vi "SETParametersToSPCdata.vi"(8 "ErrorIn":errorcluster, 10 "setFile":path=path "X:/Jannis/Abgleich/150-n scanin.set", 11 "SPCdataIn":T1={"base_adr"=0, "init"=0, "cfd_limit_low"=0.0, "cfd_limit_high"=0.0, "cfd_zc_level"=0.0, "cfd_holdoff"=0.0, "sync_zc_level"=0.0, "sync_holdoff"=0.0, "sync_threshold"=0.0, "tac_range"=0.0, "sync_freq_div"=0, "tac_gain"=0, "tac_offset"=0.0, "tac_limit_low"=0.0, "tac_limit_high"=0.0, "adc_resolution"=12, "ext_latch_delay"=0, "collect_time"=0.0, "display_time"=0.0, "repeat_time"=0.0, "stop_on_time"=0, "stop_on_ovfl"=0, "dither_range"=0, "count_incr"=0, "mem_bank"=0, "dead_time_comp"=0, "scan_control"=0, "routing_mode"=0, "tac_enable_hold"=0.0, "pci_card_no"=0, "mode"=0, "scan_size_x"=0, "scan_size_y"=0, "scan_rout_x"=0, "scan_rout_y"=0, "scan_flyback"=0, "scan_borders"=0, "scan_polarity"=0, "pixel_clock"=0, "line_compression"=0, "trigger"=0, "pixel_time"=0.0, "ext_pixclk_div"=0, "rate_count_time"=0.0, "macro_time_clk"=0, "add_select"=0, "test_eep"=0, "adc_zoom"=0, "img_size_x"=0, "img_size_y"=0, "img_rout_x"=0, "img_rout_y"=0, "xy_gain"=0, "master_clock"=0, "adc_sample_delay"=0, "detector_type"=0, "chan_enable"=0, "chan_slope"=0, "chan_spec_no"=0, "tdc_control"=0, "tdc_offset1"=0.0, "tdc_offset2"=0.0, "tdc_offset3"=0.0, "tdc_offset4"=0.0, "tdc_offset5"=0.0, "tdc_offset6"=0.0, "cfd_th5_tdc"=0.0, "cfd_th6_tdc"=0.0, "cfd_zc5_tdc"=0.0, "cfd_zc6_tdc"=0.0, "future_reserve1"=0, "future_reserve2"=0, "future_reserve3"=0, "future_reserve4"=0}) -> (0 "ErrorOut":errorcluster, 3 "SPCdataOut":T1={"base_adr"=0, "init"=0, "cfd_limit_low"=0.0, "cfd_limit_high"=0.0, "cfd_zc_level"=0.0, "cfd_holdoff"=0.0, "sync_zc_level"=0.0, "sync_holdoff"=0.0, "sync_threshold"=0.0, "tac_range"=0.0, "sync_freq_div"=0, "tac_gain"=0, "tac_offset"=0.0, "tac_limit_low"=0.0, "tac_limit_high"=0.0, "adc_resolution"=12, "ext_latch_delay"=0, "collect_time"=0.0, "display_time"=0.0, "repeat_time"=0.0, "stop_on_time"=0, "stop_on_ovfl"=0, "dither_range"=0, "count_incr"=0, "mem_bank"=0, "dead_time_comp"=0, "scan_control"=0, "routing_mode"=0, "tac_enable_hold"=0.0, "pci_card_no"=0, "mode"=0, "scan_size_x"=0, "scan_size_y"=0, "scan_rout_x"=0, "scan_rout_y"=0, "scan_flyback"=0, "scan_borders"=0, "scan_polarity"=0, "pixel_clock"=0, "line_compression"=0, "trigger"=0, "pixel_time"=0.0, "ext_pixclk_div"=0, "rate_count_time"=0.0, "macro_time_clk"=0, "add_select"=0, "test_eep"=0, "adc_zoom"=0, "img_size_x"=0, "img_size_y"=0, "img_rout_x"=0, "img_rout_y"=0, "xy_gain"=0, "master_clock"=0, "adc_sample_delay"=0, "detector_type"=0, "chan_enable"=0, "chan_slope"=0, "chan_spec_no"=0, "tdc_control"=0, "tdc_offset1"=0.0, "tdc_offset2"=0.0, "tdc_offset3"=0.0, "tdc_offset4"=0.0, "tdc_offset5"=0.0, "tdc_offset6"=0.0, "cfd_th5_tdc"=0.0, "cfd_th6_tdc"=0.0, "cfd_zc5_tdc"=0.0, "cfd_zc6_tdc"=0.0, "future_reserve1"=0, "future_reserve2"=0, "future_reserve3"=0, "future_reserve4"=0}, 4 "DecayMatrix":cluster{"Waveform Graph":sgl[]}[][](array[cluster]), 5 "ActiveModule":string[](array[string]))   [LabVIEW 2023]
doc: "This VI aids to read a full set of system parameters from a .set-file or the header of a .sdt into the SPCdata cluster. Usefull when wanting to copy all parameters established in SPCM.exe to the LV-environment.\nNote, that some parameters like <b>mode</b> are not mapped. To correctly set these parameters use SPC_set- and get_parameters.vi before calling this VI."
uses:
  SPC_Wrappers/SPC_Controls/Systparm_Kewords.ctl
  SPC_Wrappers/SPC_Controls/SPCdata.ctl
panel:
  out "String":string
  in  "Systparm_Keywords":T2
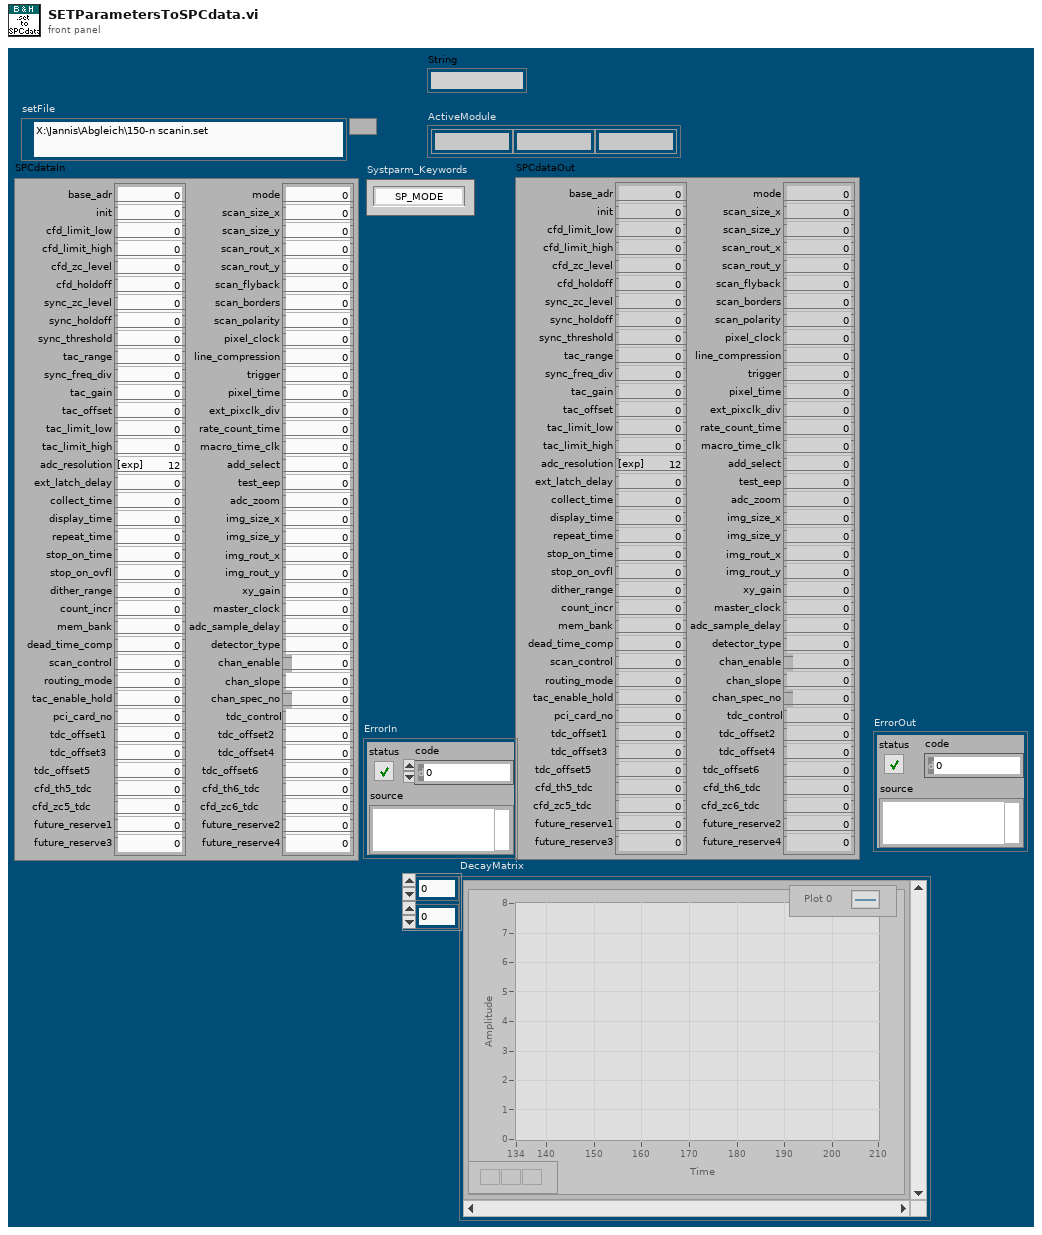
[diagram p1: front panel]
types:
  T1 = typedef "SPCdata.ctl" = cluster{"base_adr":u16, "init":i16, "cfd_limit_low":sgl, "cfd_limit_high":sgl, "cfd_zc_level":sgl, "cfd_holdoff":sgl, "sync_zc_level":sgl, "sync_holdoff":sgl, "sync_threshold":sgl, "tac_range":sgl, "sync_freq_div":i16, "tac_gain":i16, "tac_offset":sgl, "tac_limit_low":sgl, "tac_limit_high":sgl, "adc_resolution":i16, "ext_latch_delay":i16, "collect_time":sgl, "display_time":sgl, "repeat_time":sgl, "stop_on_time":i16, "stop_on_ovfl":i16, "dither_range":i16, "count_incr":i16, "mem_bank":i16, "dead_time_comp":i16, "scan_control":u16, "routing_mode":u16, "tac_enable_hold":sgl, "pci_card_no":i16, "mode":u16, "scan_size_x":u32, "scan_size_y":u32, "scan_rout_x":u32, "scan_rout_y":u32, "scan_flyback":u32, "scan_borders":u32, "scan_polarity":u16, "pixel_clock":u16, "line_compression":u16, "trigger":u16, "pixel_time":sgl, "ext_pixclk_div":u32, "rate_count_time":sgl, "macro_time_clk":i16, "add_select":i16, "test_eep":i16, "adc_zoom":i16, "img_size_x":u32, "img_size_y":u32, "img_rout_x":u32, "img_rout_y":u32, "xy_gain":i16, "master_clock":i16, "adc_sample_delay":i16, "detector_type":i16, "chan_enable":u32, "chan_slope":u32, "chan_spec_no":u32, "tdc_control":u32, "tdc_offset1":sgl, "tdc_offset2":sgl, "tdc_offset3":sgl, "tdc_offset4":sgl, "tdc_offset5":sgl, "tdc_offset6":sgl, "cfd_th5_tdc":sgl, "cfd_th6_tdc":sgl, "cfd_zc5_tdc":sgl, "cfd_zc6_tdc":sgl, "future_reserve1":u64, "future_reserve2":u64, "future_reserve3":u64, "future_reserve4":u64}
  T2 = typedef "Systparm_Kewords.ctl" = enum16{"SP_MODE", "SP_CFD_LL", "SP_CFD_LH", "SP_CFD_ZC", "SP_CFD_HF", "SP_SYN_ZC", "SP_SYN_FD", "SP_SYN_FQ", "SP_SYN_HF", "SP_TAC_R", "SP_TAC_G", "SP_TAC_OF", "SP_TAC_LL", "SP_TAC_LH", "SP_TAC_TC", "SP_TAC_TD", "SP_ADC_RE", "SP_EAL_DE", "SP_NCX", "SP_NCY", "SP_PAGE", "SP_COL_T", "SP_REP_T", "SP_DIS_T", "SP_REPEAT", "SP_STOPT", "SP_OVERFL", "SP_WL_STA", "SP_WL_STO", "SP_WL_STE", "SP_EXTST", "SP_STEPS", "SP_OFFSET", "SP_YWIN_N", "SP_XWIN_N", "SP_TWIN_N", "SP_X_EQU", "SP_Y_EQU", "SP_T_EQU", "SP_DITH", "SP_EN_INT", "SP_INCR", "SP_DAES", "SP_SPE_FN", "SP_CYCLES", "SP_DAEC", "SP_MEM_BANK", "SP_DTCOMP", "SP_SCF", "SP_POL_L", "SP_POL_F", "SP_PIX", "SP_LDIV", "SP_ACCUM", "SP_ROUT", "SP_TAC_EH", "SP_DLIM", "SP_PHOT_F", "SP_EN_DLIM", "SP_PH_BUF", "SP_FLB_Y", "SP_FLB_X", "SP_BORD_U", "SP_BORD_L", "SP_POL_P", "SP_PIX_T", "SP_PIX_CLK", "SP_TRIGGER", "SP_SCAN_X", "SP_SCAN_Y", "SP_SCAN_RX", "SP_SCAN_RY", "SP_FIF_TYP", "SP_EPX_DIV", "SP_MTCLK", "SP_ADD_SEL", "SP_SXWIN_N", "SP_SYWIN_N", "SP_SX_EQU", "SP_SY_EQU", "SP_ASAVE", "SP_ADC_ZOOM", "SP_FIF_FNO", "SP_FCYCLES", "SP_XY_GAIN", "SP_IMG_X", "SP_IMG_Y", "SP_IMG_RX", "SP_IMG_RY", "SP_MST_CLK", "SP_ADC_DE", "SP_DET_TYP", "SP_X_AXIS", "SP_CH_EN", "SP_CH_SL", "SP_CH_F1", "SP_CH_F2"}
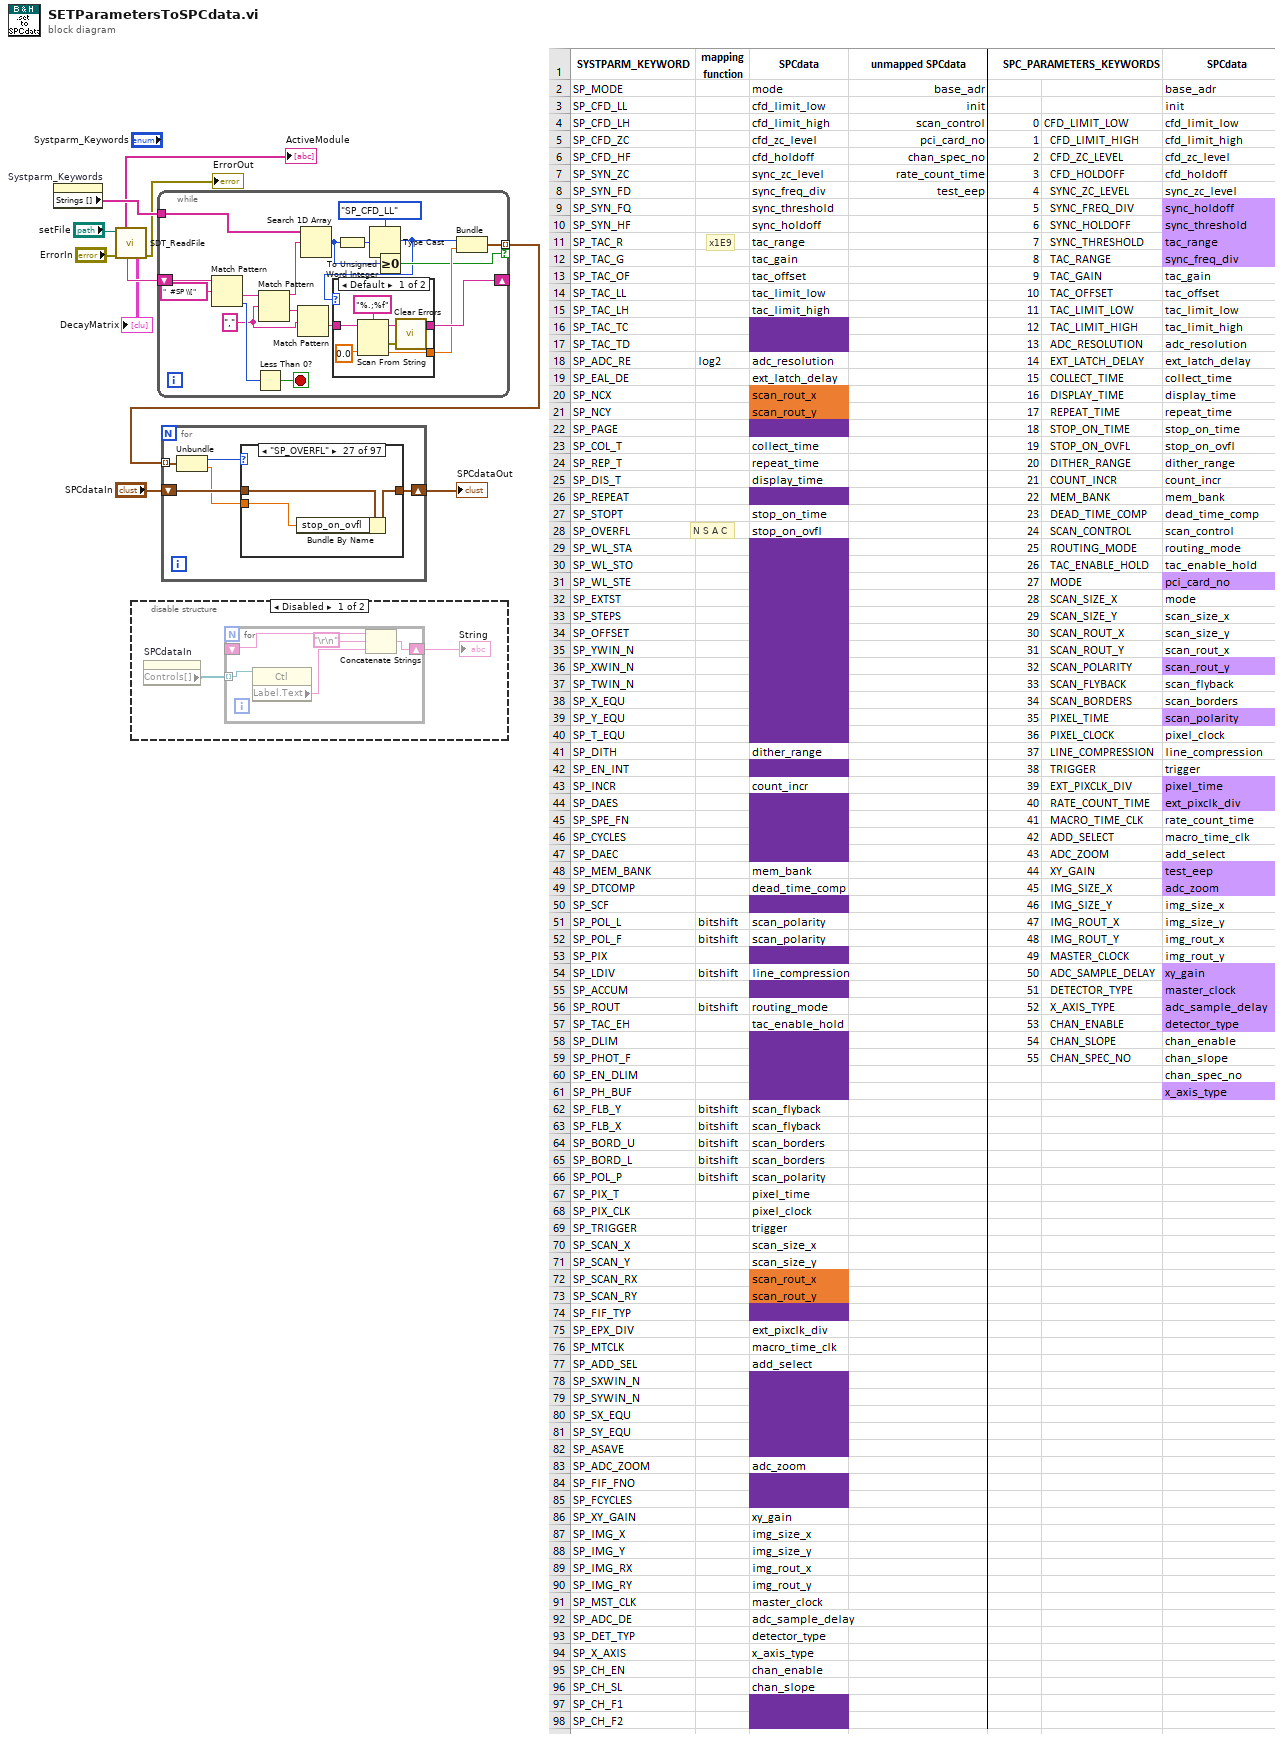
[diagram p0: block diagram]
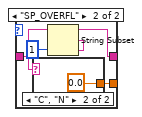
[diagram p2: hidden frame]
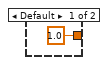
[diagram p3: hidden frame]
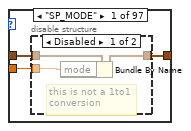
[diagram p5: hidden frame]
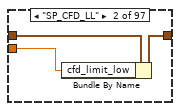
[diagram p7: hidden frame]
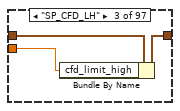
[diagram p8: hidden frame]
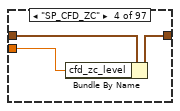
[diagram p9: hidden frame]
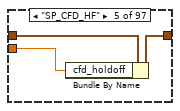
[diagram p10: hidden frame]
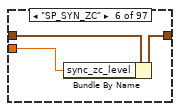
[diagram p11: hidden frame]
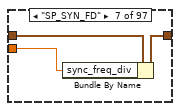
[diagram p12: hidden frame]
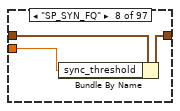
[diagram p13: hidden frame]
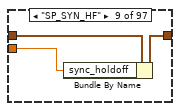
[diagram p14: hidden frame]
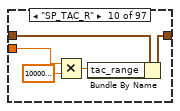
[diagram p15: hidden frame]
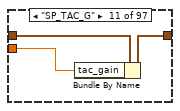
[diagram p16: hidden frame]
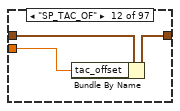
[diagram p17: hidden frame]
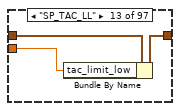
[diagram p18: hidden frame]
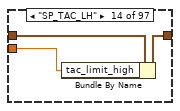
[diagram p19: hidden frame]
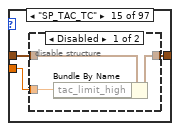
[diagram p20: hidden frame]
diagram:
  # "N S A C"
  # "x1E9"
  n1 = property on="Systparm_Keywords" class="Enum (strict)"() -> ("Strings []"=w6:string[])  [unwired: 2 in, 2 out]
  n2 = call "SDT_ReadFile.vi"("error in"="ErrorIn", "sdtFile"="setFile") -> ("error out"=→"ErrorOut":errorcluster, "DecayMatrix"=→"DecayMatrix":cluster{"Waveform Graph":sgl[]}[][], "SetUp"=w7:string, "ActiveModule"=→"ActiveModule":string[])  [unwired: 2 in, 4 out]
  n3 = disable-structure shown="Disabled" {
    frame Disabled {
      n4 = property on="SPCdataIn" class="Clust (strict)"() -> ("Controls[]"=w12:refnum<vi>[])  [unwired: 2 in, 2 out]
      n5 = for {
        tunnel: w12 -> [w17] mode=indexing
        shift-right: [w15] -> w11
        shift-left: _ -> [w14]
        n6 = property class="Ctl"(reference=w17) -> ("Label.Text"=w16:string)  [unwired: 1 in, 2 out]
        n7 = Concatenate Strings(w14, "\r\n", w16) -> (w15:string)
      }
      "String" <- w11
    }
    frame Enabled {
    }
  }
  n8 = while {
    shift-right: [w27] -> _
    shift-left: w7 -> [w35]
    tunnel: w6 -> [w25]
    tunnel: [w22] -> w5 mode=indexing if=w20
    stop <- w32 stop-if-true
    w29 = "," ("regular expression")
    n9 = Match Pattern(string=w35, regular expression="  #SP \\[") -> (after substring=w33:string, offset past match=w31:i32)  [unwired: 1 in, 2 out]
    n10 = Less Than 0?(x=w31) -> (x < 0?=w32:bool)
    n11 = Match Pattern(string=w33, regular expression=w29) -> (before substring=w26:string, after substring=w30:string)  [unwired: 1 in, 2 out]
    n12 = Match Pattern(string=w30, regular expression=w29) -> (after substring=w28:string)  [unwired: 1 in, 3 out]
    n13 = Search 1D Array(1D array=w25, element=w26) -> (index of element=w21:i32)  [unwired: 1 in]
    n14 = To Unsigned Word Integer(number=w21) -> (unsigned 16bit integer=w19:u16)
    n15 = Type Cast(type=Systparm_Kewords."SP_CFD_LL" ("Systparm_Keywords"), x=w19) -> (*(type *) &x=w18:T2)
    n16 = case shown="Default" w18 {
      tunnel: w28 -> [w41 w43]
      tunnel: [w38 w43] -> w27
      tunnel: [w37 w42] -> w23
      frame Default {
        n17 = Scan From String(format string="%.;%f", input string=w41, default 1=sgl 0.0 ("Value")) -> (remaining string=w38:string, error out=w36:errorcluster, output 1=w37:sgl)  [unwired: 2 in, 1 out]
        n18 = call <vilib>:"Clear Errors.vi"("error in (no error)"=w36) -> ()  [unwired: 5 in, 2 out]
      }
      frame "SP_OVERFL" {
        n19 = String Subset(string=w43, length (rest)=1 ("length (rest)")) -> (substring=w44:string)  [unwired: 1 in]
        n20 = case shown="\"C\", \"N\"" w44 {
          tunnel: [sgl 1.0 ("Value") sgl 0.0 ("Value")] -> w42
          frame Default {
          }
          frame "C", "N" {
          }
        }
      }
    }
    n21 = Greater Or Equal To 0?(x=w21) -> (x >= 0?=w20:bool)
    n22 = Bundle("Systparm_Keywords"=w18, "Value"=w23) -> (w22:cluster{"Systparm_Keywords":T2, "Value":sgl})  [unwired: 1 in]
  }
  n23 = for {
    shift-right: [w51] -> w9
    shift-left: "SPCdataIn" -> [w52]
    tunnel: w5 -> [w50] mode=indexing
    n24 = Unbundle(w50) -> ("Systparm_Keywords"=w49:T2, "Value"=w48:sgl)
    n25 = case shown="\"SP_OVERFL\"" w49 {
      tunnel: w52 -> [w54 w62 w65 w68 w71 w74 w77 w80 w83 w88 w91 w94 w97 w100 w103 w110 w118 w121 w124 w127 w130 w137 w140 w143 w146 w153 w156 w159 w166 w173 w180 w187 w194 w201 w208 w215 w222 w229 w236 w243 w246 w253 w256 w263 w270 w277 w284 w287 w290 w301 w311 w315 w324 w327 w336 w339 w342 w349 w356 w363 w375 w382 w391 w398 w408 w411 w414 w417 w420 w423 w426 w429 w432 w439 w442 w445 w448 w455 w462 w469 w476 w483 w486 w493 w500 w503 w506 w509 w512 w515 w518 w521 w524 w527 w530 w533 w540]
      tunnel: [w55 w61 w64 w67 w70 w73 w76 w79 w82 w87 w90 w93 w96 w99 w102 w109 w117 w120 w123 w126 w129 w136 w139 w142 w145 w152 w155 w158 w165 w172 w179 w186 w193 w200 w207 w214 w221 w228 w235 w242 w245 w252 w255 w262 w269 w276 w283 w286 w289 w302 w312 w314 w323 w326 w335 w338 w341 w348 w355 w362 w376 w383 w392 w399 w409 w412 w415 w418 w421 w424 w427 w430 w433 w440 w443 w446 w449 w456 w463 w470 w477 w484 w487 w494 w501 w504 w507 w510 w513 w516 w519 w522 w525 w528 w531 w534 w541] -> w51
      tunnel: w48 -> [w53 w60 w63 w66 w69 w72 w75 w78 w81 w86 w89 w92 w95 w98 w101 w108 w116 w119 w122 w125 w128 w135 w138 w141 w144 w151 w154 w157 w164 w171 w178 w185 w192 w199 w206 w213 w220 w227 w234 w241 w244 w251 w254 w261 w268 w275 w282 w285 w288 w298 w306 w313 w322 w325 w334 w337 w340 w347 w354 w361 w372 w377 w386 w393 w403 w410 w413 w416 w419 w422 w425 w428 w431 w438 w441 w444 w447 w454 w461 w468 w475 w482 w485 w492 w499 w502 w505 w508 w511 w514 w517 w520 w523 w526 w529 w532 w539]
      frame "SP_MODE" {
        n26 = disable-structure shown="Disabled" {
          disable-tunnel: [w58 w59] -> w55
          disable-tunnel: w54 -> [w57 w59]
          disable-tunnel: w53 -> [w56 _]
          frame Disabled {
            # "this is not a 1to1\nconversion"
            n27 = Bundle By Name(cluster=w57, "mode"=w56) -> (w58:T1)
          }
          frame Enabled {
          }
        }
      }
      frame "SP_CFD_LL" {
        n28 = Bundle By Name(cluster=w62, "cfd_limit_low"=w60) -> (w61:T1)
      }
      frame "SP_CFD_LH" {
        n29 = Bundle By Name(cluster=w65, "cfd_limit_high"=w63) -> (w64:T1)
      }
      frame "SP_CFD_ZC" {
        n30 = Bundle By Name(cluster=w68, "cfd_zc_level"=w66) -> (w67:T1)
      }
      frame "SP_CFD_HF" {
        n31 = Bundle By Name(cluster=w71, "cfd_holdoff"=w69) -> (w70:T1)
      }
      frame "SP_SYN_ZC" {
        n32 = Bundle By Name(cluster=w74, "sync_zc_level"=w72) -> (w73:T1)
      }
      frame "SP_SYN_FD" {
        n33 = Bundle By Name(cluster=w77, "sync_freq_div"=w75) -> (w76:T1)
      }
      frame "SP_SYN_FQ" {
        n34 = Bundle By Name(cluster=w80, "sync_threshold"=w78) -> (w79:T1)
      }
      frame "SP_SYN_HF" {
        n35 = Bundle By Name(cluster=w83, "sync_holdoff"=w81) -> (w82:T1)
      }
      frame "SP_TAC_R" {
        n36 = Multiply(x=w86, y=sgl 1000000000.0) -> (x*y=w85:sgl)
        n37 = Bundle By Name(cluster=w88, "tac_range"=w85) -> (w87:T1)
      }
      frame "SP_TAC_G" {
        n38 = Bundle By Name(cluster=w91, "tac_gain"=w89) -> (w90:T1)
      }
      frame "SP_TAC_OF" {
        n39 = Bundle By Name(cluster=w94, "tac_offset"=w92) -> (w93:T1)
      }
      frame "SP_TAC_LL" {
        n40 = Bundle By Name(cluster=w97, "tac_limit_low"=w95) -> (w96:T1)
      }
      frame "SP_TAC_LH" {
        n41 = Bundle By Name(cluster=w100, "tac_limit_high"=w98) -> (w99:T1)
      }
      frame "SP_TAC_TC" {
        n42 = disable-structure shown="Disabled" {
          disable-tunnel: w103 -> [w106 w107]
          disable-tunnel: [w105 w107] -> w102
          disable-tunnel: w101 -> [w104 _]
          frame Disabled {
            n43 = Bundle By Name(cluster=w106, "tac_limit_high"=w104) -> (w105:T1)
          }
          frame Enabled {
          }
        }
      }
      frame "SP_TAC_TD" {
        n44 = disable-structure shown="Enabled" {
          disable-tunnel: w110 -> [w113 w114]
          disable-tunnel: [w112 w114] -> w109
          disable-tunnel: w108 -> [w111 _]
          frame Disabled {
            n45 = Bundle By Name(cluster=w113, "sync_holdoff"=w111) -> (w112:T1)
          }
          frame Enabled {
          }
        }
      }
      frame "SP_ADC_RE" {
        n46 = Logarithm Base 2(1:w116) -> (0:w115:sgl)
        n47 = Bundle By Name(cluster=w118, "adc_resolution"=w115) -> (w117:T1)
      }
      frame "SP_EAL_DE" {
        n48 = Bundle By Name(cluster=w121, "ext_latch_delay"=w119) -> (w120:T1)
      }
      frame "SP_NCX" {
        n49 = Bundle By Name(cluster=w124, "scan_rout_x"=w122) -> (w123:T1)
      }
      frame "SP_NCY" {
        n50 = Bundle By Name(cluster=w127, "scan_rout_y"=w125) -> (w126:T1)
      }
      frame "SP_PAGE" {
        n51 = disable-structure shown="Disabled" {
          disable-tunnel: w130 -> [w133 w134]
          disable-tunnel: [w132 w134] -> w129
          disable-tunnel: w128 -> [w131 _]
          frame Disabled {
            n52 = Bundle By Name(cluster=w133, "scan_rout_y"=w131) -> (w132:T1)
          }
          frame Enabled {
          }
        }
      }
      frame "SP_COL_T" {
        n53 = Bundle By Name(cluster=w137, "collect_time"=w135) -> (w136:T1)
      }
      frame "SP_REP_T" {
        n54 = Bundle By Name(cluster=w140, "repeat_time"=w138) -> (w139:T1)
      }
      frame "SP_DIS_T" {
        n55 = Bundle By Name(cluster=w143, "display_time"=w141) -> (w142:T1)
      }
      frame "SP_REPEAT" {
        n56 = disable-structure shown="Disabled" {
          disable-tunnel: w146 -> [w149 w150]
          disable-tunnel: [w148 w150] -> w145
          disable-tunnel: w144 -> [w147 _]
          frame Disabled {
            n57 = Bundle By Name(cluster=w149, "repeat_time"=w147) -> (w148:T1)
          }
          frame Enabled {
          }
        }
      }
      frame "SP_STOPT" {
        n58 = Bundle By Name(cluster=w153, "stop_on_time"=w151) -> (w152:T1)
      }
      frame "SP_OVERFL" {
        n59 = Bundle By Name(cluster=w156, "stop_on_ovfl"=w154) -> (w155:T1)
      }
      frame "SP_WL_STA" {
        n60 = disable-structure shown="Disabled" {
          disable-tunnel: w159 -> [w162 w163]
          disable-tunnel: [w161 w163] -> w158
          disable-tunnel: w157 -> [w160 _]
          frame Disabled {
            n61 = Bundle By Name(cluster=w162, "stop_on_ovfl"=w160) -> (w161:T1)
          }
          frame Enabled {
          }
        }
      }
      frame "SP_WL_STO" {
        n62 = disable-structure shown="Disabled" {
          disable-tunnel: w166 -> [w169 w170]
          disable-tunnel: [w168 w170] -> w165
          disable-tunnel: w164 -> [w167 _]
          frame Disabled {
            n63 = Bundle By Name(cluster=w169, "stop_on_ovfl"=w167) -> (w168:T1)
          }
          frame Enabled {
          }
        }
      }
      frame "SP_WL_STE" {
        n64 = disable-structure shown="Disabled" {
          disable-tunnel: w173 -> [w176 w177]
          disable-tunnel: [w175 w177] -> w172
          disable-tunnel: w171 -> [w174 _]
          frame Disabled {
            n65 = Bundle By Name(cluster=w176, "stop_on_ovfl"=w174) -> (w175:T1)
          }
          frame Enabled {
          }
        }
      }
      frame "SP_EXTST" {
        n66 = disable-structure shown="Disabled" {
          disable-tunnel: w180 -> [w183 w184]
          disable-tunnel: [w182 w184] -> w179
          disable-tunnel: w178 -> [w181 _]
          frame Disabled {
            n67 = Bundle By Name(cluster=w183, "stop_on_ovfl"=w181) -> (w182:T1)
          }
          frame Enabled {
          }
        }
      }
      frame "SP_STEPS" {
        n68 = disable-structure shown="Disabled" {
          disable-tunnel: w187 -> [w190 w191]
          disable-tunnel: [w189 w191] -> w186
          disable-tunnel: w185 -> [w188 _]
          frame Disabled {
            n69 = Bundle By Name(cluster=w190, "stop_on_ovfl"=w188) -> (w189:T1)
          }
          frame Enabled {
          }
        }
      }
      frame "SP_OFFSET" {
        n70 = disable-structure shown="Disabled" {
          disable-tunnel: w194 -> [w197 w198]
          disable-tunnel: [w196 w198] -> w193
          disable-tunnel: w192 -> [w195 _]
          frame Disabled {
            n71 = Bundle By Name(cluster=w197, "stop_on_ovfl"=w195) -> (w196:T1)
          }
          frame Enabled {
          }
        }
      }
      frame "SP_YWIN_N" {
        n72 = disable-structure shown="Disabled" {
          disable-tunnel: w201 -> [w204 w205]
          disable-tunnel: [w203 w205] -> w200
          disable-tunnel: w199 -> [w202 _]
          frame Disabled {
            n73 = Bundle By Name(cluster=w204, "stop_on_ovfl"=w202) -> (w203:T1)
          }
          frame Enabled {
          }
        }
      }
      frame "SP_XWIN_N" {
        n74 = disable-structure shown="Disabled" {
          disable-tunnel: w208 -> [w211 w212]
          disable-tunnel: [w210 w212] -> w207
          disable-tunnel: w206 -> [w209 _]
          frame Disabled {
            n75 = Bundle By Name(cluster=w211, "stop_on_ovfl"=w209) -> (w210:T1)
          }
          frame Enabled {
          }
        }
      }
      frame "SP_TWIN_N" {
        n76 = disable-structure shown="Disabled" {
          disable-tunnel: w215 -> [w218 w219]
          disable-tunnel: [w217 w219] -> w214
          disable-tunnel: w213 -> [w216 _]
          frame Disabled {
            n77 = Bundle By Name(cluster=w218, "stop_on_ovfl"=w216) -> (w217:T1)
          }
          frame Enabled {
          }
        }
      }
      frame "SP_X_EQU" {
        n78 = disable-structure shown="Disabled" {
          disable-tunnel: w222 -> [w225 w226]
          disable-tunnel: [w224 w226] -> w221
          disable-tunnel: w220 -> [w223 _]
          frame Disabled {
            n79 = Bundle By Name(cluster=w225, "stop_on_ovfl"=w223) -> (w224:T1)
          }
          frame Enabled {
          }
        }
      }
      frame "SP_Y_EQU" {
        n80 = disable-structure shown="Disabled" {
          disable-tunnel: w229 -> [w232 w233]
          disable-tunnel: [w231 w233] -> w228
          disable-tunnel: w227 -> [w230 _]
          frame Disabled {
            n81 = Bundle By Name(cluster=w232, "stop_on_ovfl"=w230) -> (w231:T1)
          }
          frame Enabled {
          }
        }
      }
      frame "SP_T_EQU" {
        n82 = disable-structure shown="Disabled" {
          disable-tunnel: w236 -> [w239 w240]
          disable-tunnel: [w238 w240] -> w235
          disable-tunnel: w234 -> [w237 _]
          frame Disabled {
            n83 = Bundle By Name(cluster=w239, "stop_on_ovfl"=w237) -> (w238:T1)
          }
          frame Enabled {
          }
        }
      }
      frame "SP_DITH" {
        n84 = Bundle By Name(cluster=w243, "dither_range"=w241) -> (w242:T1)
      }
      frame "SP_EN_INT" {
        n85 = disable-structure shown="Disabled" {
          disable-tunnel: w246 -> [w249 w250]
          disable-tunnel: [w248 w250] -> w245
          disable-tunnel: w244 -> [w247 _]
          frame Disabled {
            n86 = Bundle By Name(cluster=w249, "dither_range"=w247) -> (w248:T1)
          }
          frame Enabled {
          }
        }
      }
      frame "SP_INCR" {
        n87 = Bundle By Name(cluster=w253, "count_incr"=w251) -> (w252:T1)
      }
      frame "SP_DAES" {
        n88 = disable-structure shown="Disabled" {
          disable-tunnel: w256 -> [w259 w260]
          disable-tunnel: [w258 w260] -> w255
          disable-tunnel: w254 -> [w257 _]
          frame Disabled {
            n89 = Bundle By Name(cluster=w259, "count_incr"=w257) -> (w258:T1)
          }
          frame Enabled {
          }
        }
      }
      frame "SP_SPE_FN" {
        n90 = disable-structure shown="Disabled" {
          disable-tunnel: w263 -> [w266 w267]
          disable-tunnel: [w265 w267] -> w262
          disable-tunnel: w261 -> [w264 _]
          frame Disabled {
            n91 = Bundle By Name(cluster=w266, "count_incr"=w264) -> (w265:T1)
          }
          frame Enabled {
          }
        }
      }
      frame "SP_CYCLES" {
        n92 = disable-structure shown="Disabled" {
          disable-tunnel: w270 -> [w273 w274]
          disable-tunnel: [w272 w274] -> w269
          disable-tunnel: w268 -> [w271 _]
          frame Disabled {
            n93 = Bundle By Name(cluster=w273, "count_incr"=w271) -> (w272:T1)
          }
          frame Enabled {
          }
        }
      }
      frame "SP_DAEC" {
        n94 = disable-structure shown="Disabled" {
          disable-tunnel: w277 -> [w280 w281]
          disable-tunnel: [w279 w281] -> w276
          disable-tunnel: w275 -> [w278 _]
          frame Disabled {
            n95 = Bundle By Name(cluster=w280, "count_incr"=w278) -> (w279:T1)
          }
          frame Enabled {
          }
        }
      }
      frame "SP_MEM_BANK" {
        n96 = Bundle By Name(cluster=w284, "mem_bank"=w282) -> (w283:T1)
      }
      frame "SP_DTCOMP" {
        n97 = Bundle By Name(cluster=w287, "dead_time_comp"=w285) -> (w286:T1)
      }
      frame "SP_SCF" {
        n98 = disable-structure shown="Disabled" {
          disable-tunnel: w290 -> [w293 w294]
          disable-tunnel: [w292 w294] -> w289
          disable-tunnel: w288 -> [w291 _]
          frame Disabled {
            n99 = Bundle By Name(cluster=w293, "mem_bank"=w291) -> (w292:T1)
          }
          frame Enabled {
          }
        }
      }
      frame "SP_POL_L" {
        n100 = To Unsigned Word Integer(number=w298) -> (unsigned 16bit integer=w295:u16)
        n101 = Unbundle By Name(w301) -> ("scan_polarity"=w300:u16)
        n102 = And(x=w300, y=u16 65534) -> (x .and. y?=w296:u16)
        n103 = Or(x=w296, y=w295) -> (x .or. y?=w297:u16)
        n104 = Bundle By Name(cluster=w301, "scan_polarity"=w297) -> (w302:T1)
      }
      frame "SP_POL_F" {
        n105 = To Unsigned Word Integer(number=w306) -> (unsigned 16bit integer=w303:u16)
        n106 = Unbundle By Name(w311) -> ("scan_polarity"=w310:u16)
        n107 = Logical Shift(y=u16 1 ("x .and. y?"), x=w303) -> (x << y=w305:u16)
        n108 = And(x=w310, y=u16 65533) -> (x .and. y?=w307:u16)
        n109 = Or(x=w307, y=w305) -> (x .or. y?=w308:u16)
        n110 = Bundle By Name(cluster=w311, "scan_polarity"=w308) -> (w312:T1)
      }
      frame "SP_PIX" {
        n111 = disable-structure shown="Disabled" {
          disable-tunnel: w315 -> [w318 w319]
          disable-tunnel: [w317 w319] -> w314
          disable-tunnel: w313 -> [w316 _]
          frame Disabled {
            n112 = Bundle By Name(cluster=w318, "mem_bank"=w316) -> (w317:T1)
          }
          frame Enabled {
          }
        }
      }
      frame "SP_LDIV" {
        n113 = Logical Shift(y=w322, x=i16 1 ("y")) -> (x << y=w321:i16)
        n114 = Bundle By Name(cluster=w324, "line_compression"=w321) -> (w323:T1)
      }
      frame "SP_ACCUM" {
        n115 = disable-structure shown="Disabled" {
          disable-tunnel: w327 -> [w330 w331]
          disable-tunnel: [w329 w331] -> w326
          disable-tunnel: w325 -> [w328 _]
          frame Disabled {
            n116 = Bundle By Name(cluster=w330, "pixel_clock"=w328) -> (w329:T1)
          }
          frame Enabled {
          }
        }
      }
      frame "SP_ROUT" {
        n117 = Logical Shift(y=i16 6, x=w334) -> (x << y=w333:u32)
        n118 = Bundle By Name(cluster=w336, "routing_mode"=w333) -> (w335:T1)
      }
      frame "SP_TAC_EH" {
        n119 = Bundle By Name(cluster=w339, "tac_enable_hold"=w337) -> (w338:T1)
      }
      frame "SP_DLIM" {
        n120 = disable-structure shown="Disabled" {
          disable-tunnel: w342 -> [w345 w346]
          disable-tunnel: [w344 w346] -> w341
          disable-tunnel: w340 -> [w343 _]
          frame Disabled {
            n121 = Bundle By Name(cluster=w345, "tac_enable_hold"=w343) -> (w344:T1)
          }
          frame Enabled {
          }
        }
      }
      frame "SP_PHOT_F" {
        n122 = disable-structure shown="Disabled" {
          disable-tunnel: w349 -> [w352 w353]
          disable-tunnel: [w351 w353] -> w348
          disable-tunnel: w347 -> [w350 _]
          frame Disabled {
            n123 = Bundle By Name(cluster=w352, "tac_enable_hold"=w350) -> (w351:T1)
          }
          frame Enabled {
          }
        }
      }
      frame "SP_EN_DLIM" {
        n124 = disable-structure shown="Disabled" {
          disable-tunnel: w356 -> [w359 w360]
          disable-tunnel: [w358 w360] -> w355
          disable-tunnel: w354 -> [w357 _]
          frame Disabled {
            n125 = Bundle By Name(cluster=w359, "tac_enable_hold"=w357) -> (w358:T1)
          }
          frame Enabled {
          }
        }
      }
      frame "SP_PH_BUF" {
        n126 = disable-structure shown="Disabled" {
          disable-tunnel: w363 -> [w366 w367]
          disable-tunnel: [w365 w367] -> w362
          disable-tunnel: w361 -> [w364 _]
          frame Disabled {
            n127 = Bundle By Name(cluster=w366, "tac_enable_hold"=w364) -> (w365:T1)
          }
          frame Enabled {
          }
        }
      }
      frame "SP_FLB_Y" {
        n128 = Unbundle By Name(w375) -> ("scan_flyback"=w374:u32)
        n129 = Logical Shift(y=i16 16, x=w372) -> (x << y=w370:u32)
        n130 = And(x=w374, y=u32 65535) -> (x .and. y?=w368:u32)
        n131 = Or(x=w368, y=w370) -> (x .or. y?=w369:u32)
        n132 = Bundle By Name(cluster=w375, "scan_flyback"=w369) -> (w376:T1)
      }
      frame "SP_FLB_X" {
        n133 = Unbundle By Name(w382) -> ("scan_flyback"=w381:u32)
        n134 = And(x=w381, y=u32 4294901760) -> (x .and. y?=w378:u32)
        n135 = Or(x=w378, y=w377) -> (x .or. y?=w379:i32)
        n136 = Bundle By Name(cluster=w382, "scan_flyback"=w379) -> (w383:T1)
      }
      frame "SP_BORD_U" {
        n137 = Unbundle By Name(w391) -> ("scan_borders"=w390:u32)
        n138 = Logical Shift(y=i16 16, x=w386) -> (x << y=w385:u32)
        n139 = And(x=w390, y=u32 65535) -> (x .and. y?=w387:u32)
        n140 = Or(x=w387, y=w385) -> (x .or. y?=w388:u32)
        n141 = Bundle By Name(cluster=w391, "scan_borders"=w388) -> (w392:T1)
      }
      frame "SP_BORD_L" {
        n142 = Unbundle By Name(w398) -> ("scan_borders"=w397:u32)
        n143 = And(x=w397, y=u32 4294901760) -> (x .and. y?=w394:u32)
        n144 = Or(x=w394, y=w393) -> (x .or. y?=w395:i32)
        n145 = Bundle By Name(cluster=w398, "scan_borders"=w395) -> (w399:T1)
      }
      frame "SP_POL_P" {
        n146 = To Unsigned Word Integer(number=w403) -> (unsigned 16bit integer=w400:u16)
        n147 = Unbundle By Name(w408) -> ("scan_polarity"=w407:u16)
        n148 = Logical Shift(y=i16 2, x=w400) -> (x << y=w402:u16)
        n149 = And(x=w407, y=u16 65531) -> (x .and. y?=w404:u16)
        n150 = Or(x=w404, y=w402) -> (x .or. y?=w405:u16)
        n151 = Bundle By Name(cluster=w408, "scan_polarity"=w405) -> (w409:T1)
      }
      frame "SP_PIX_T" {
        n152 = Bundle By Name(cluster=w411, "pixel_time"=w410) -> (w412:T1)
      }
      frame "SP_PIX_CLK" {
        n153 = Bundle By Name(cluster=w414, "pixel_clock"=w413) -> (w415:T1)
      }
      frame "SP_TRIGGER" {
        n154 = Bundle By Name(cluster=w417, "trigger"=w416) -> (w418:T1)
      }
      frame "SP_SCAN_X" {
        n155 = Bundle By Name(cluster=w420, "scan_size_x"=w419) -> (w421:T1)
      }
      frame "SP_SCAN_Y" {
        n156 = Bundle By Name(cluster=w423, "scan_size_y"=w422) -> (w424:T1)
      }
      frame "SP_SCAN_RX" {
        n157 = Bundle By Name(cluster=w426, "scan_rout_x"=w425) -> (w427:T1)
      }
      frame "SP_SCAN_RY" {
        n158 = Bundle By Name(cluster=w429, "scan_rout_y"=w428) -> (w430:T1)
      }
      frame "SP_FIF_TYP" {
        n159 = disable-structure shown="Disabled" {
          disable-tunnel: [w436 w437] -> w433
          disable-tunnel: w432 -> [w435 w437]
          disable-tunnel: w431 -> [w434 _]
          frame Disabled {
            n160 = Bundle By Name(cluster=w435, "scan_rout_y"=w434) -> (w436:T1)
          }
          frame Enabled {
          }
        }
      }
      frame "SP_EPX_DIV" {
        n161 = Bundle By Name(cluster=w439, "ext_pixclk_div"=w438) -> (w440:T1)
      }
      frame "SP_MTCLK" {
        n162 = Bundle By Name(cluster=w442, "macro_time_clk"=w441) -> (w443:T1)
      }
      frame "SP_ADD_SEL" {
        n163 = Bundle By Name(cluster=w445, "add_select"=w444) -> (w446:T1)
      }
      frame "SP_SXWIN_N" {
        n164 = disable-structure shown="Disabled" {
          disable-tunnel: [w452 w453] -> w449
          disable-tunnel: w448 -> [w451 w453]
          disable-tunnel: w447 -> [w450 _]
          frame Disabled {
            n165 = Bundle By Name(cluster=w451, "add_select"=w450) -> (w452:T1)
          }
          frame Enabled {
          }
        }
      }
      frame "SP_SYWIN_N" {
        n166 = disable-structure shown="Disabled" {
          disable-tunnel: [w459 w460] -> w456
          disable-tunnel: w455 -> [w458 w460]
          disable-tunnel: w454 -> [w457 _]
          frame Disabled {
            n167 = Bundle By Name(cluster=w458, "add_select"=w457) -> (w459:T1)
          }
          frame Enabled {
          }
        }
      }
      frame "SP_SX_EQU" {
        n168 = disable-structure shown="Disabled" {
          disable-tunnel: [w466 w467] -> w463
          disable-tunnel: w462 -> [w465 w467]
          disable-tunnel: w461 -> [w464 _]
          frame Disabled {
            n169 = Bundle By Name(cluster=w465, "add_select"=w464) -> (w466:T1)
          }
          frame Enabled {
          }
        }
      }
      frame "SP_SY_EQU" {
        n170 = disable-structure shown="Disabled" {
          disable-tunnel: [w473 w474] -> w470
          disable-tunnel: w469 -> [w472 w474]
          disable-tunnel: w468 -> [w471 _]
          frame Disabled {
            n171 = Bundle By Name(cluster=w472, "add_select"=w471) -> (w473:T1)
          }
          frame Enabled {
          }
        }
      }
      frame "SP_ASAVE" {
        n172 = disable-structure shown="Disabled" {
          disable-tunnel: [w480 w481] -> w477
          disable-tunnel: w476 -> [w479 w481]
          disable-tunnel: w475 -> [w478 _]
          frame Disabled {
            n173 = Bundle By Name(cluster=w479, "add_select"=w478) -> (w480:T1)
          }
          frame Enabled {
          }
        }
      }
      frame "SP_ADC_ZOOM" {
        n174 = Bundle By Name(cluster=w483, "adc_zoom"=w482) -> (w484:T1)
      }
      frame "SP_FIF_FNO" {
        n175 = disable-structure shown="Disabled" {
          disable-tunnel: [w490 w491] -> w487
          disable-tunnel: w486 -> [w489 w491]
          disable-tunnel: w485 -> [w488 _]
          frame Disabled {
            n176 = Bundle By Name(cluster=w489, "adc_zoom"=w488) -> (w490:T1)
          }
          frame Enabled {
          }
        }
      }
      frame "SP_FCYCLES" {
        n177 = disable-structure shown="Disabled" {
          disable-tunnel: [w497 w498] -> w494
          disable-tunnel: w493 -> [w496 w498]
          disable-tunnel: w492 -> [w495 _]
          frame Disabled {
            n178 = Bundle By Name(cluster=w496, "adc_zoom"=w495) -> (w497:T1)
          }
          frame Enabled {
          }
        }
      }
      frame "SP_XY_GAIN" {
        n179 = Bundle By Name(cluster=w500, "xy_gain"=w499) -> (w501:T1)
      }
      frame "SP_IMG_X" {
        n180 = Bundle By Name(cluster=w503, "img_size_x"=w502) -> (w504:T1)
      }
      frame "SP_IMG_Y" {
        n181 = Bundle By Name(cluster=w506, "img_size_y"=w505) -> (w507:T1)
      }
      frame "SP_IMG_RX" {
        n182 = Bundle By Name(cluster=w509, "img_rout_x"=w508) -> (w510:T1)
      }
      frame "SP_IMG_RY" {
        n183 = Bundle By Name(cluster=w512, "img_rout_y"=w511) -> (w513:T1)
      }
      frame "SP_MST_CLK" {
        n184 = Bundle By Name(cluster=w515, "master_clock"=w514) -> (w516:T1)
      }
      frame "SP_ADC_DE" {
        n185 = Bundle By Name(cluster=w518, "adc_sample_delay"=w517) -> (w519:T1)
      }
      frame "SP_DET_TYP" {
        n186 = Bundle By Name(cluster=w521, "detector_type"=w520) -> (w522:T1)
      }
      frame "SP_X_AXIS" {
        n187 = Bundle By Name(cluster=w524, "tdc_control"=w523) -> (w525:T1)
      }
      frame "SP_CH_EN" {
        n188 = Bundle By Name(cluster=w527, "chan_enable"=w526) -> (w528:T1)
      }
      frame "SP_CH_SL" {
        n189 = Bundle By Name(cluster=w530, "chan_slope"=w529) -> (w531:T1)
      }
      frame "SP_CH_F1" {
        n190 = disable-structure shown="Enabled" {
          disable-tunnel: [w537 w538] -> w534
          disable-tunnel: w533 -> [w536 w538]
          disable-tunnel: w532 -> [w535 _]
          frame Disabled {
            n191 = Bundle By Name(cluster=w536, "chan_slope"=w535) -> (w537:T1)
          }
          frame Enabled {
          }
        }
      }
      frame "SP_CH_F2" {
        n192 = disable-structure shown="Disabled" {
          disable-tunnel: [w544 w545] -> w541
          disable-tunnel: w540 -> [w543 w545]
          disable-tunnel: w539 -> [w542 _]
          frame Disabled {
            n193 = Bundle By Name(cluster=w543, "chan_slope"=w542) -> (w544:T1)
          }
          frame Enabled {
          }
        }
      }
    }
  }
  "SPCdataOut" <- w9
